vi "adam-digital-inputs.vi"(0 "VISA Refnum in":refnum<visa-resource-name>, 1 "Chassis Settings":T2, 2 "sample?":bool, 5 "Current DI State":T1, 9 "chassis-slot":i32, 11 "error in (no error)":errorcluster, 12 "cmd-in":string, 13 "ack char":string) -> (4 "VISA Refnum out":refnum<visa-resource-name>, 6 "New DI State":T1, 8 "cmd-out":string, 10 "acknowledge char":string, 14 "cmd aknowledged":bool, 15 "error out":errorcluster)   [LabVIEW 2024]
uses:
  controls/adam-5000-serial-settings.ctl
  controls/digitial-input-cluster.ctl
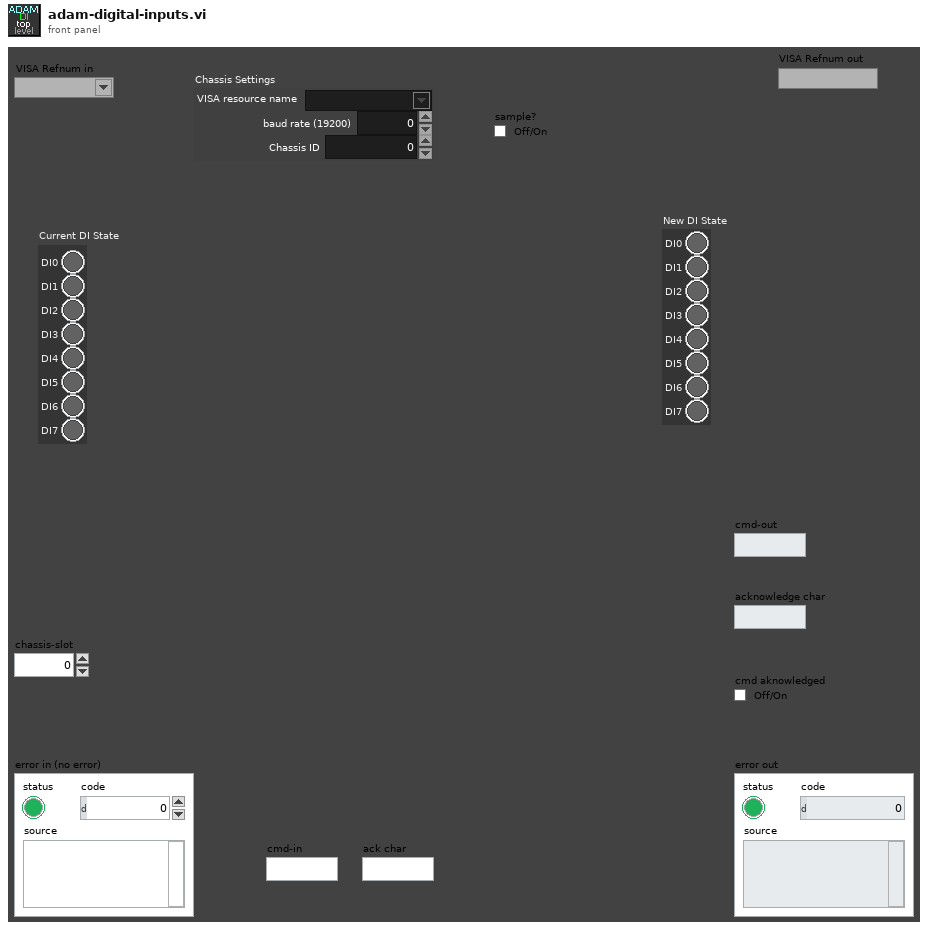
[diagram p1: front panel]
types:
  T1 = typedef "digitial-input-cluster.ctl" = cluster{"DI0":bool, "DI1":bool, "DI2":bool, "DI3":bool, "DI4":bool, "DI5":bool, "DI6":bool, "DI7":bool}
  T2 = typedef "adam-5000-serial-settings.ctl" = cluster{"VISA resource name":refnum<visa-resource-name>, "baud rate (19200)":u32, "Chassis ID":u8}
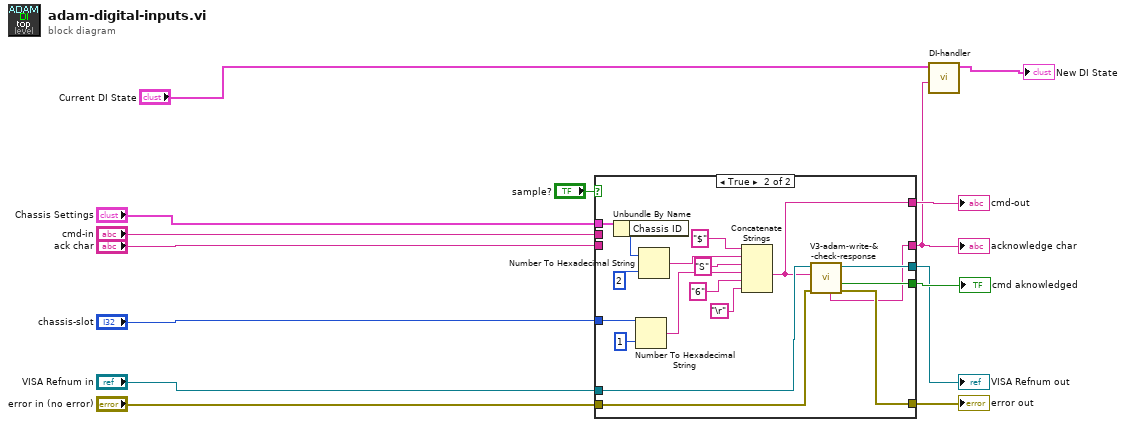
[diagram p0: block diagram]
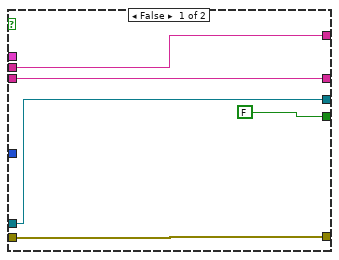
[diagram p2: hidden frame]
diagram:
  n1 = case shown="True" "sample?" {
    tunnel: "Chassis Settings" -> [_ w37]
    tunnel: "chassis-slot" -> [_ w32]
    tunnel: "VISA Refnum in" -> [w19 w28]
    tunnel: "error in (no error)" -> [w17 w27]
    tunnel: [w17 w26] -> w9
    tunnel: [w19 w25] -> w10
    tunnel: [FALSE ("cmd aknowledged") w24] -> w12
    tunnel: [w16 w20] -> w4
    tunnel: "ack char" -> [w16 _]
    tunnel: [w15 w23] -> w13
    tunnel: "cmd-in" -> [w15 _]
    frame False {
    }
    frame True {
      n2 = Unbundle By Name(w37) -> ("Chassis ID"=w36:u8)
      n3 = Number To Hexadecimal String(1:i16 1 ("width (-)"), 2:w32) -> (0:w30:string)
      n4 = Number To Hexadecimal String(1:i16 2 ("width (-)"), 2:w36) -> (0:w34:string)
      n5 = Concatenate Strings("$" ("string"), w34, "S" ("string"), w30, "6" ("string"), "\r") -> (w23:string)
      n6 = call "V3-adam-write-&-check-response.vi"("error in (no error)"=w27, "write buffer"=w23, "VISA resource name"=w28) -> ("error out"=w26:errorcluster, "cmd aknowledged"=w24:bool, "VISA resource name out"=w25:refnum<visa-resource-name>, "read buffer"=w20:string)  [unwired: 4 in, 1 out]
    }
  }
  "cmd-out" <- w13
  "cmd aknowledged" <- w12
  "acknowledge char" <- w4
  "VISA Refnum out" <- w10
  "error out" <- w9
  n7 = call "DI-handler.vi"("hex integer string in"=w4, "Current DI State"="Current DI State") -> ("New DI State"=→"New DI State":T1)  [unwired: 8 in, 1 out]
